vi "VenomDriveEncoderConverter.vi"(2 "Mode":enum16{"Count -> Inches", "Inches -> Count"}(ring), 3 "Input":dbl) -> (1 "Output":dbl)   [LabVIEW 2018]
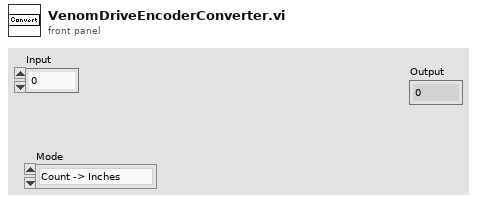
[diagram p1: front panel]
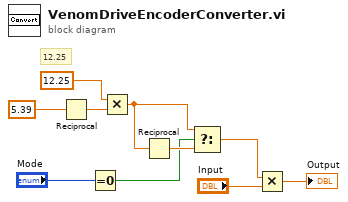
[diagram p0: block diagram]
diagram:
  # "12.25"
  n1 = Reciprocal(x=5.39) -> (1/x=w3:dbl)
  n2 = Equal To 0?(x="Mode") -> (x = 0?=w6:bool)
  n3 = Multiply(x=12.25, y=w3) -> (x*y=w2:dbl)
  n4 = Reciprocal(x=w2) -> (1/x=w10:dbl)
  n5 = Select(t=w2, s=w6, f=w10) -> (s? t:f=w1:dbl)
  n6 = Multiply(x=w1, y="Input") -> (x*y=→"Output":dbl)
